vi "FrameworkHL.vi"(7 "StandardRequests":refnum<event-registration>, 10 "Message Queue":refnum<class "RQMHMessageQueue.lvclass">, 11 "JQMHModule in":refnum<class "RQMHModule.lvclass">) -> ()   [LabVIEW 2024, in "RQMHModule.lvclass"]
doc: "Helper loop for framework tasks"
uses:
  RQMHModule.lvclass
  ModQueue/RQMHMessageQueue.lvclass
  StandardRequests.ctl
  InitialiseArgs.ctl
  Reply.ctl
  StopEventArgs.ctl
  Show Front Panel--Args.ctl
  Hide Front Panel.ctl
  Show Block Diagram.ctl
  Hide Block Diagram--Args.ctl
  ModQueue/RQMHMessageQueue.lvclass/RQMHMessageQueue.ctl
  RQMHModule.lvclass/RQMHModule.ctl
  ModQueue/Delacor_lib_QMH_Enqueue Message (Single).vi
  Shared/RQMHShared.lvlib
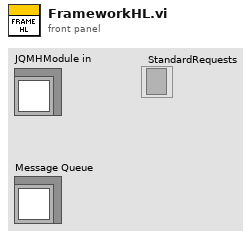
[diagram p1: front panel]
types:
  T1 = enum32{"Invalid", "Standard", "Closed", "Hidden", "Minimized", "Maximized"}
  T2 = typedef "RQMHModule.lvclass/InitialiseArgs.ctl" = cluster{"null":bool}
  T3 = typedef "RQMHModule.lvclass/Reply.ctl" = cluster{"Expects Reply":bool, "Reply":refnum<notifier>}
  T4 = typedef "RQMHModule.lvclass/Show Front Panel--Args.ctl" = variant
  T5 = typedef "RQMHModule.lvclass/Show Block Diagram.ctl" = bool
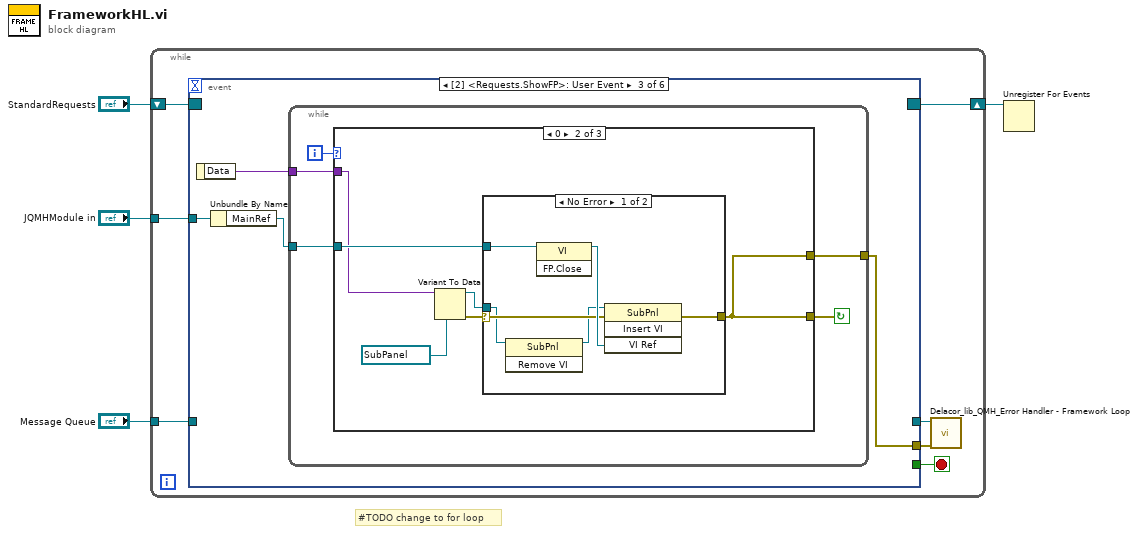
[diagram p0: block diagram]
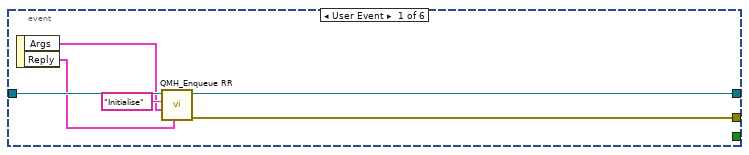
[diagram p2: hidden frame]
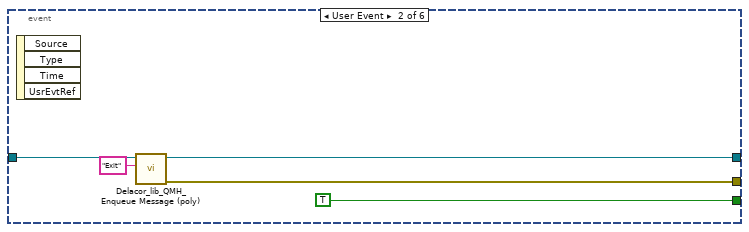
[diagram p3: hidden frame]
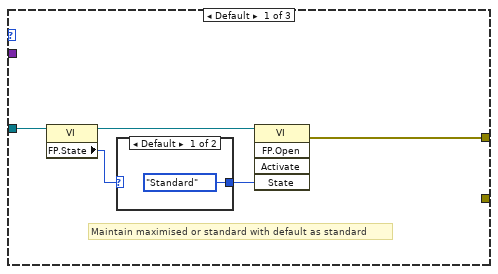
[diagram p4: hidden frame]
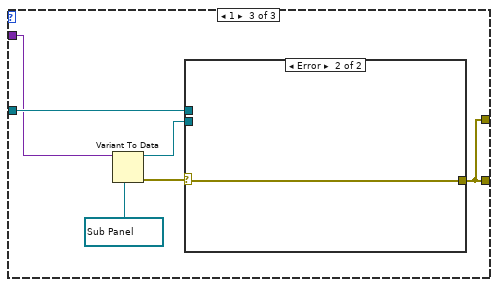
[diagram p7: hidden frame]
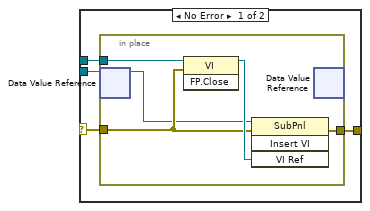
[diagram p8: hidden frame]
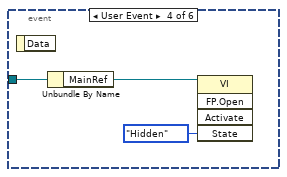
[diagram p9: hidden frame]
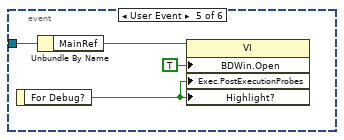
[diagram p10: hidden frame]
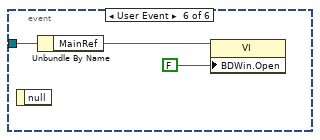
[diagram p11: hidden frame]
diagram:
  # "#TODO change to for loop"
  n1 = while {
    shift-right: [w11] -> w4
    shift-left: "StandardRequests" -> [w5]
    tunnel: "Message Queue" -> [w10]
    tunnel: "JQMHModule in" -> [w6]
    stop <- w7 stop-if-true
    n2 = event shown="[2] <Requests.ShowFP>: User Event" {
      selector: w5 -> [_ _ _ _ _ _]
      dyn-events: [_ _ _ _ _ _] -> w11
      timeout: _ -> [_ _ _ _ _ _]
      tunnel: w10 -> [w17 w20 _ _ _ _]
      tunnel: [w16 w19 _ _ _ _] -> w9
      tunnel: [w15 w18 w23 _ _ _] -> w8
      tunnel: [_ TRUE _ _ _ _] -> w7
      tunnel: w6 -> [_ _ w26 w70 w74 w77]
      event User Event {
        n3 = event-data() -> ("Args"=w13:T2, "Reply"=w12:T3)  [unwired: 1 in]
        n4 = call "QMH_Enqueue RR.vi"("Reply"=w12, "Message Data"=w13, "Message"="Initialise", "Message Queue in"=w17) -> ("error out"=w15:errorcluster, "Message Queue out"=w16:refnum<class "RQMHMessageQueue.lvclass">)  [unwired: 6 in]
      }
      event User Event {
        n5 = event-data() -> ()  [unwired: 1 in, 4 out]
        n6 = call-poly "Delacor_lib_QMH_Enqueue Message (poly).vi"("Message"="Exit", "Message Queue in"=w20) -> ("error out"=w18:errorcluster, "Message Queue out"=w19:refnum<class "RQMHMessageQueue.lvclass">)  [unwired: 8 in]
      }
      event User Event {
        n7 = event-data() -> ("Data"=w24:T4)  [unwired: 1 in]
        n8 = Unbundle By Name(w26) -> ("MainRef"=w25:refnum<vi>)
        n9 = while {
          tunnel: w25 -> [w30]
          tunnel: [w28] -> w23
          tunnel: w24 -> [w27]
          i -> [w31]
          stop <- w29 continue-if-true
          n10 = case shown="0" w31 {
            tunnel: w30 -> [w36 w44 w57]
            tunnel: [_ w43 w56] -> w29
            tunnel: w27 -> [_ w40 w55]
            tunnel: [w35 w43 w56] -> w28
            frame Default {
              # "Maintain maximised or standard with default as standard"
              n11 = property class="VI"(reference=w36) -> (reference out=w34:refnum<vi>, "FP.State"=w33:T1)  [unwired: 1 in, 1 out]
              n12 = case shown="Default" w33 {
                selector: w33 -> [_ w38]
                tunnel: [T1."Standard" ("FP.State") w38] -> w32
                frame Default {
                }
                frame "Standard", "Maximized" {
                }
              }
              n13 = invoke class="VI" method="FP.Open"(reference=w34, "State"=w32) -> (error out=w35:errorcluster)  [unwired: 3 in, 4 out]
            }
            frame 0 {
              n14 = Variant To Data(type=refnum<vi> refnum ("Sub Panel"), Variant=w40) -> (data=w41:refnum<vi>, error out=w42:errorcluster)  [unwired: 1 in]
              n15 = case shown="No Error" w42 {
                selector: w42 -> [w47 w51]
                tunnel: w41 -> [w45 _]
                tunnel: w44 -> [w50 _]
                tunnel: [w48 w51] -> w43
                frame No Error {
                  n16 = invoke class="SubPnl" method="Remove VI"(reference=w45) -> (reference out=w46:refnum<vi>)  [unwired: 2 in, 2 out]
                  n17 = invoke class="VI" method="FP.Close"(reference=w50) -> (reference out=w49:refnum<vi>)  [unwired: 2 in, 2 out]
                  n18 = invoke class="SubPnl" method="Insert VI"(reference=w46, error in=w47, "VI Ref"=w49) -> (error out=w48:errorcluster)  [unwired: 1 in, 3 out]
                }
                frame Error {
                }
              }
            }
            frame 1 {
              n19 = Variant To Data(type=refnum<data-value> refnum ("data value reference"), Variant=w55) -> (data=w52:refnum<data-value>, error out=w53:errorcluster)  [unwired: 1 in]
              n20 = case shown="Error" w53 {
                selector: w53 -> [w59 w67]
                tunnel: w57 -> [w61 _]
                tunnel: [w60 w67] -> w56
                tunnel: w52 -> [w58 _]
                frame No Error {
                  n21 = in-place {
                    in-place-border: w61 -> [w66]
                    in-place-border: [w64] -> w60
                    in-place-border: w59 -> [w63]
                    n22 = in-place-dvr #1(w58) -> (w62:refnum<vi>)  [unwired: 1 out]
                    n23 = invoke class="VI" method="FP.Close"(reference=w66, error in=w63) -> (reference out=w65:refnum<vi>)  [unwired: 1 in, 2 out]
                    n24 = invoke class="SubPnl" method="Insert VI"(reference=w62, error in=w63, "VI Ref"=w65) -> (error out=w64:errorcluster)  [unwired: 1 in, 3 out]
                    n25 = in-place-dvr #1() -> ()  [unwired: 1 in, 2 out]
                  }
                }
                frame Error {
                }
              }
            }
          }
        }
      }
      event User Event {
        n26 = event-data() -> ()  [unwired: 1 in, 1 out]
        n27 = Unbundle By Name(w70) -> ("MainRef"=w69:refnum<vi>)
        n28 = invoke class="VI" method="FP.Open"(reference=w69, "State"=T1."Hidden") -> ()  [unwired: 3 in, 5 out]
      }
      event User Event {
        n29 = event-data() -> ("For Debug?"=w72:T5)  [unwired: 1 in]
        n30 = Unbundle By Name(w74) -> ("MainRef"=w73:refnum<vi>)
        n31 = property class="VI"(reference=w73, "BDWin.Open"=TRUE ("Block Diagram Window:Open"), "Exec.PostExecutionProbes"=w72, "Highlight?"=w72) -> ()  [unwired: 1 in, 2 out]
      }
      event User Event {
        n32 = event-data() -> ()  [unwired: 1 in, 1 out]
        n33 = Unbundle By Name(w77) -> ("MainRef"=w76:refnum<vi>)
        n34 = property class="VI"(reference=w76, "BDWin.Open"=FALSE ("Block Diagram Window:Open")) -> ()  [unwired: 1 in, 2 out]
      }
    }
    n35 = call-dynamic "Delacor_lib_QMH_Error Handler - Framework Loop.vi"("error in"=w8, "Message Queue in"=w9) -> ()  [unwired: 8 in, 2 out]
  }
  n36 = Unregister For Events(event registration refnum=w4) -> ()  [unwired: 1 in, 1 out]
